vi "WDT Number of Waveform Samples EXT.vi"(8 "error in (no error)":errorcluster, 11 "waveform in":waveform(ext)) -> (0 "error out":errorcluster, 2 "number of samples":i32, 3 "waveform out":waveform(ext))   [LabVIEW 2011]
doc: "Returns the number of data elements in the waveform. You must manually select the polymorphic instance you want to use."
panel:
  in  "Waveform ERROR":waveform(ext)={"t0"=timestamp(0 s since 1904-01-01), "dt"=0.0, "Y"=[]}
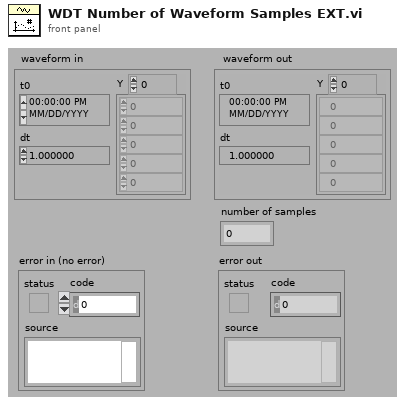
[diagram p1: front panel]
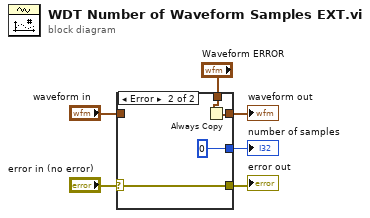
[diagram p0: block diagram]
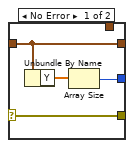
[diagram p2: hidden frame]
diagram:
  n1 = case shown="Error" "error in (no error)" {
    selector: "error in (no error)" -> [w7 w12]
    tunnel: "waveform in" -> [w8 _]
    tunnel: [w8 w11] -> w5
    tunnel: [w9 0] -> w6
    tunnel: "Waveform ERROR" -> [_ w13]
    tunnel: [w7 w12] -> w2
    frame No Error {
      n2 = Unbundle By Name(w8) -> ("Y"=w10:ext[])
      n3 = Array Size(array=w10) -> (size(s)=w9:i32)
    }
    frame Error {
      # "Incoming Error"
      n4 = Always Copy(1:w13) -> (0:w11:waveform(ext))
    }
  }
  "number of samples" <- w6
  "waveform out" <- w5
  "error out" <- w2
